vi "ShopPlane.vi"() -> ()   [LabVIEW 2013]
uses:
  InfoTable.lvclass
  ShopBase.lvclass
panel:
  in  "正在营业":bool
  in  "位置":string
  out "布尔":bool
  in  "OK":bool
  in  "名称":string
  out "?":i32(listbox)
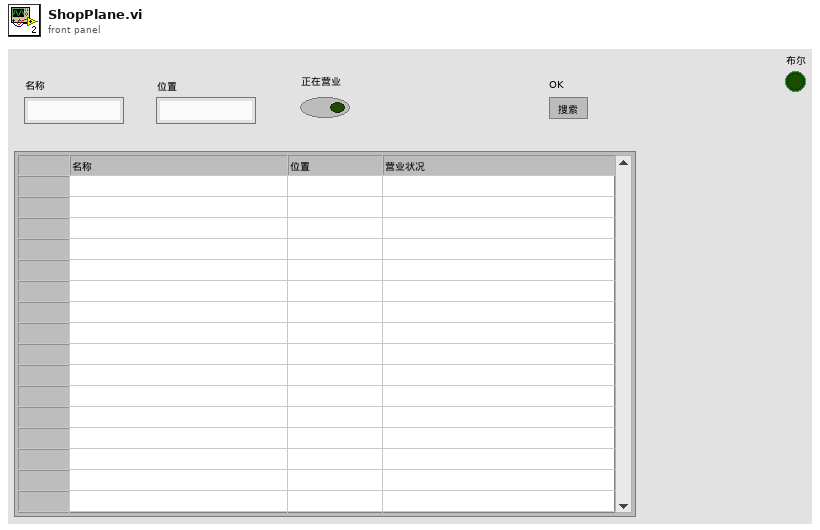
[diagram p1: front panel]
types:
  T1 = cluster{"ID":dbl, "商店名称":string, "商店位置":string, "是否营业":bool, "菜品ID":dbl[]}[]
  T2 = cluster{"ID":dbl, "商店名称":string, "商店位置":string, "是否营业":bool, "菜品ID":dbl[]}
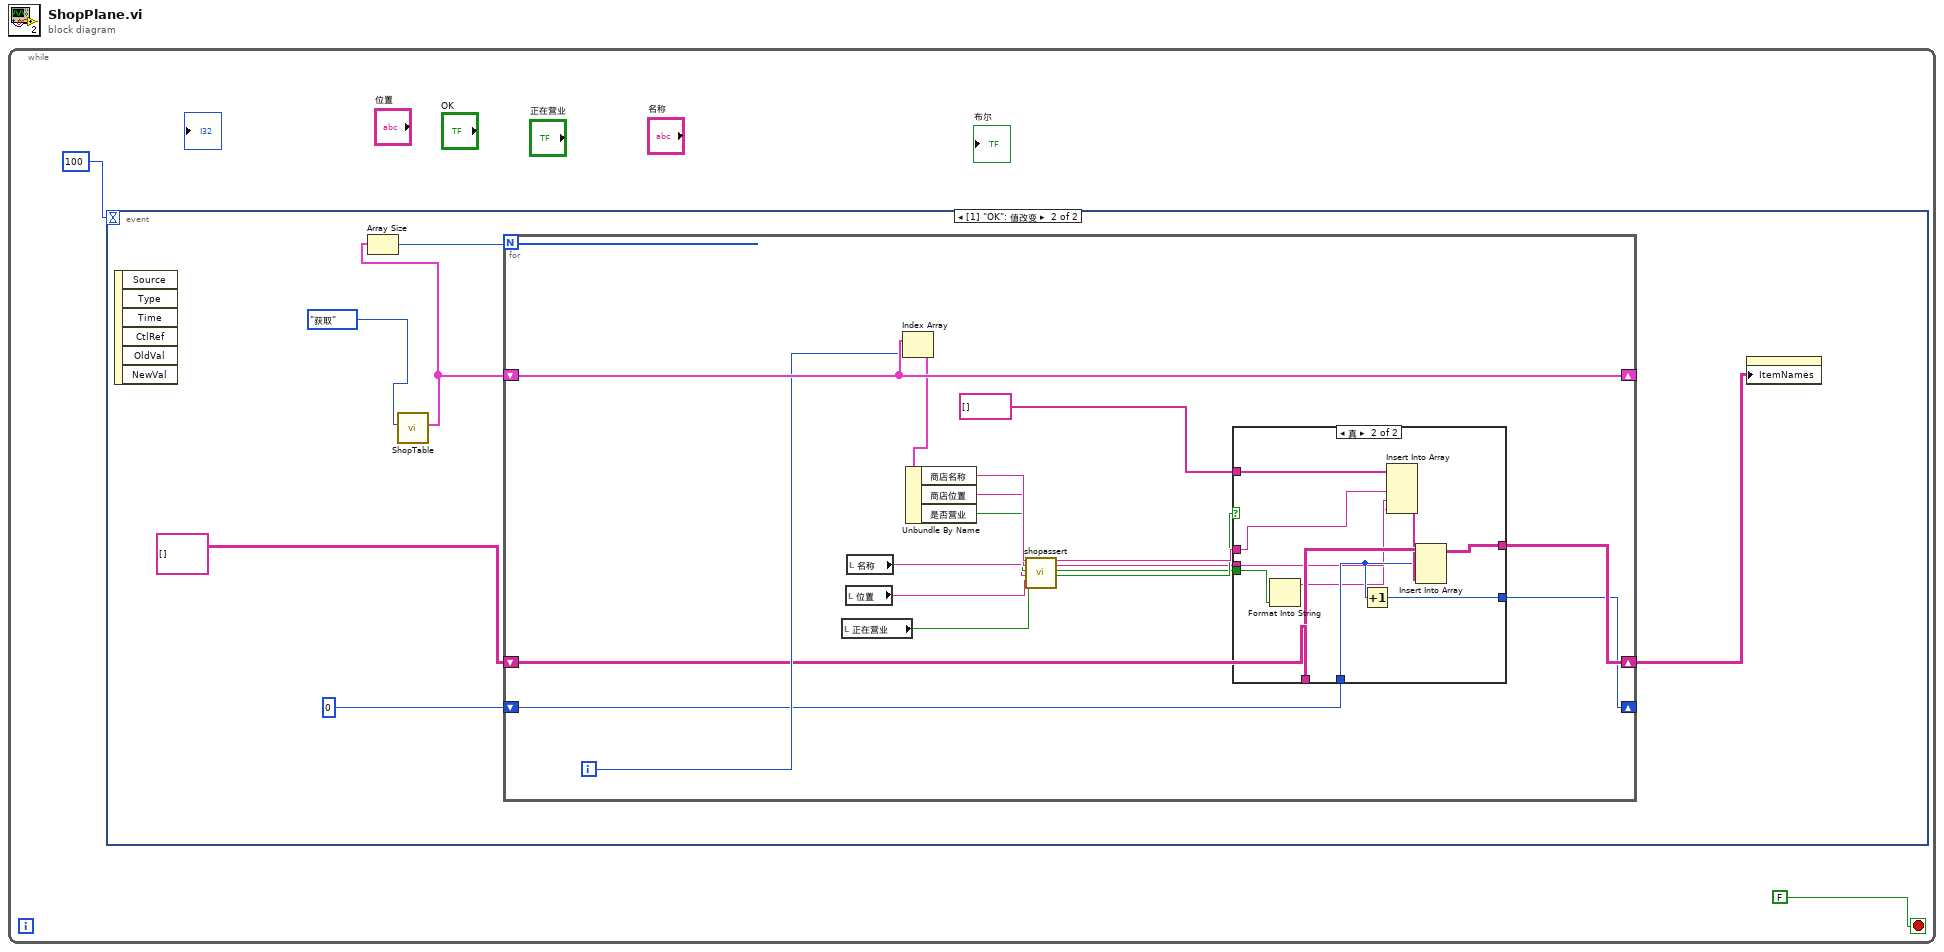
[diagram p0: block diagram]
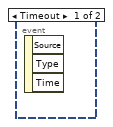
[diagram p2: hidden frame]
diagram:
  n1 = while {
    stop <- FALSE stop-if-true
    n2 = event shown="[1] \"OK\": 值改变" {
      selector: _ -> [_ _]
      dyn-events: _ -> [_ _]
      timeout: 100 -> [_ _]
      event Timeout {
        n3 = event-data() -> ()  [unwired: 1 in, 3 out]
      }
      event "OK": Value Change {
        n4 = event-data() -> ()  [unwired: 1 in, 6 out]
        n5 = call "ShopTable.vi"("枚举"=enum16{"保存", "获取", "清空", "插入", "删除", "查询"}."获取") -> ("数组 2"=w3:T1)  [unwired: 4 in, 2 out]
        n6 = Array Size(array=w3) -> (size(s)=w7:i32)
        n7 = for {
          N: w7 -> [_]
          shift-right: [w26] -> _
          shift-left: w3 -> [w26]
          shift-right: [w22] -> w6
          shift-left: string[][] [] ("数组") -> [w23]
          shift-right: [w19] -> _
          shift-left: 0 -> [w20]
          i -> [w24]
          n8 = local read "正在营业"() -> (w13:bool)
          n9 = local read "位置"() -> (w14:string)
          n10 = local read "名称"() -> (w15:string)
          n11 = Index Array(array=w26, index=w24) -> (element=w25:T2)
          n12 = Unbundle By Name(w25) -> ("商店名称"=w18:string, "商店位置"=w17:string, "是否营业"=w16:bool)
          n13 = call "shopassert.vi"("名称"=w18, "位置"=w17, "正在营业"=w16, "名称 4"=w15, "位置 2"=w14, "正在营业 2"=w13) -> ("名称 5"=w12:string, "位置 3"=w10:string, "正在营业 3"=w9:bool, "正确？"=w11:bool)  [unwired: 10 in]
          n14 = case shown="真" w11 {
            tunnel: w23 -> [w28 w38]
            tunnel: [w28 w34] -> w22
            tunnel: string[] [] -> [_ w37]
            tunnel: w12 -> [_ w36]
            tunnel: w20 -> [w27 w33]
            tunnel: [w27 w32] -> w19
            tunnel: w10 -> [_ w31]
            tunnel: w9 -> [_ w30]
            frame False {
            }
            frame True {
              n15 = Format Into String(w30) -> (resulting string=w29:string)  [unwired: 3 in, 1 out]
              n16 = Increment(x=w33) -> (x+1=w32:i32)
              n17 = Insert Into Array(array=w37, new element #1=w36, new element #2=w31, new element #3=w29) -> (w35:string[])  [unwired: 1 in]
              n18 = Insert Into Array(array=w38, index (row)=w33, new element=w35) -> (w34:string[][])  [unwired: 1 in]
            }
          }
        }
        n19 = property class="MCListbox (严格)"("ItemNames"=w6) -> ()  [unwired: 2 in, 2 out]
      }
    }
  }
